vi "_ISV Calibration.vi"(6 "Progress Bar":refnum<vi>, 8 "Error In":errorcluster, 11 "ADC Channel Calibration In":string[][](table)) -> (0 "Error Out":errorcluster, 1 "aborted":bool, 2 "ADC Table":T1[](array[typedef]), 3 "ADC Channel Calibration Out":string[][](table))   [LabVIEW 2018]
uses:
  Type/_RT Configuration 2.ctl
  Type/_RT Command.ctl
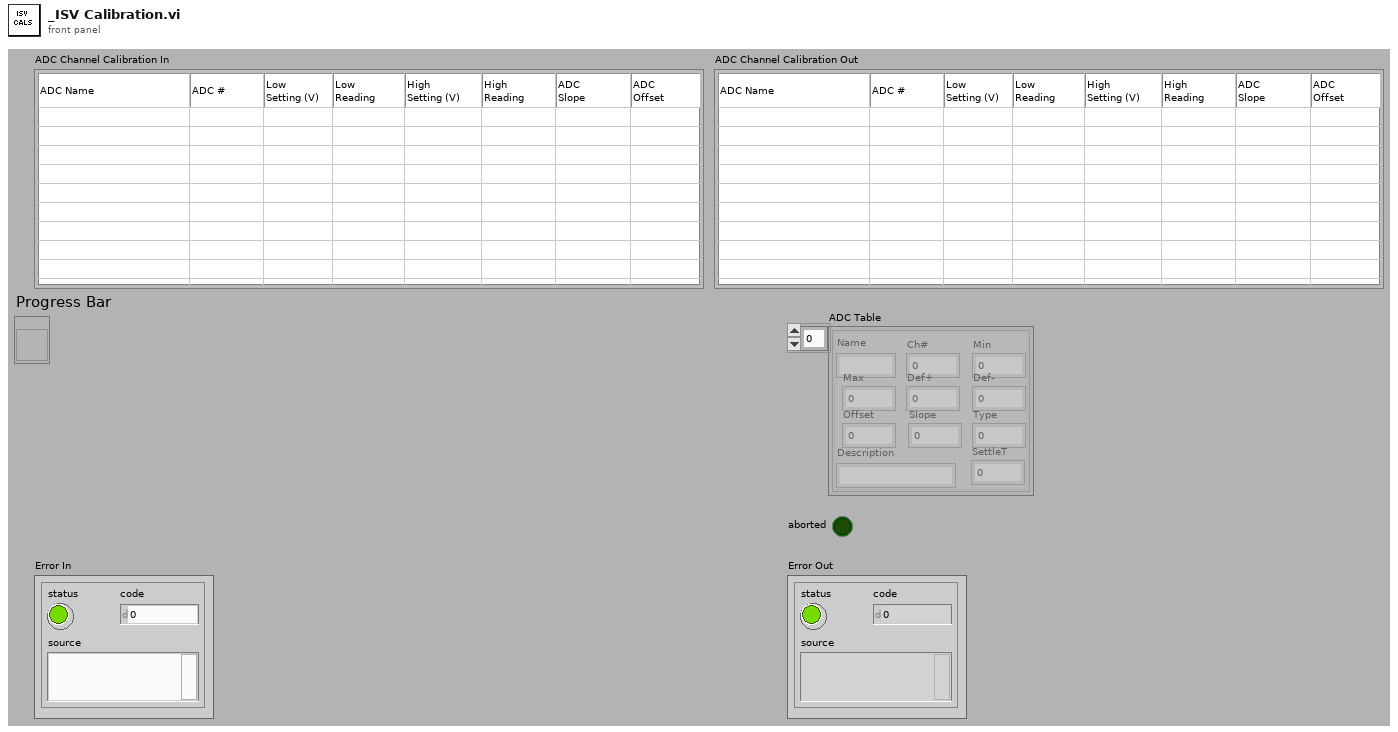
[diagram p1: front panel]
types:
  T1 = typedef "_RT Configuration 2.ctl" = cluster{"Name":string, "Ch#":u8, "Min":dbl, "Max":dbl, "Def+":dbl, "Def-":dbl, "Offset":dbl, "Slope":dbl, "Type":u8, "Description":string, "SettleT":dbl}
  T2 = typedef "_RT Command.ctl" = enum16{"xml Start Run", "xml Start Actual Run", "xml Stop Run", "xml Runtime Update", "xml Get Status", "xml Get Table", "xml Set Table", "xml Get Configuration", "xml System Status", "xml Set LC Input Logic", "xml Get Data", "xml Get Info", "Start", "StartActualRun", "Stop", "Runtime Update", "Get Data", "Get Info", "Get Status", "Get Param", "Get Config", "Get Table", "Read ADC", "Set Oscillator", "Update Config", "Update Table", "Set All Pol", "Set Pol and DC", "Set Max Mass", "Toggle RP", "Toggle EL", "Set PIC", "Initialize Turbo", "Send Turbo Comm", "Close Turbo", "P1", "P2", "P3", "Send Serial", "Set LC Out", "Get LC In", "Read VAC", "Test Table", "Toggle Power", "Get Startup", "Set Startup", "Get ADC Table", "Set ADC Table", "Get Brief Status", "Get Detail Status", "Auxiliary Update", "Set CC Logics", "Test Channel", "Set CC Input Logics", "Ignore Error", "invalid"}
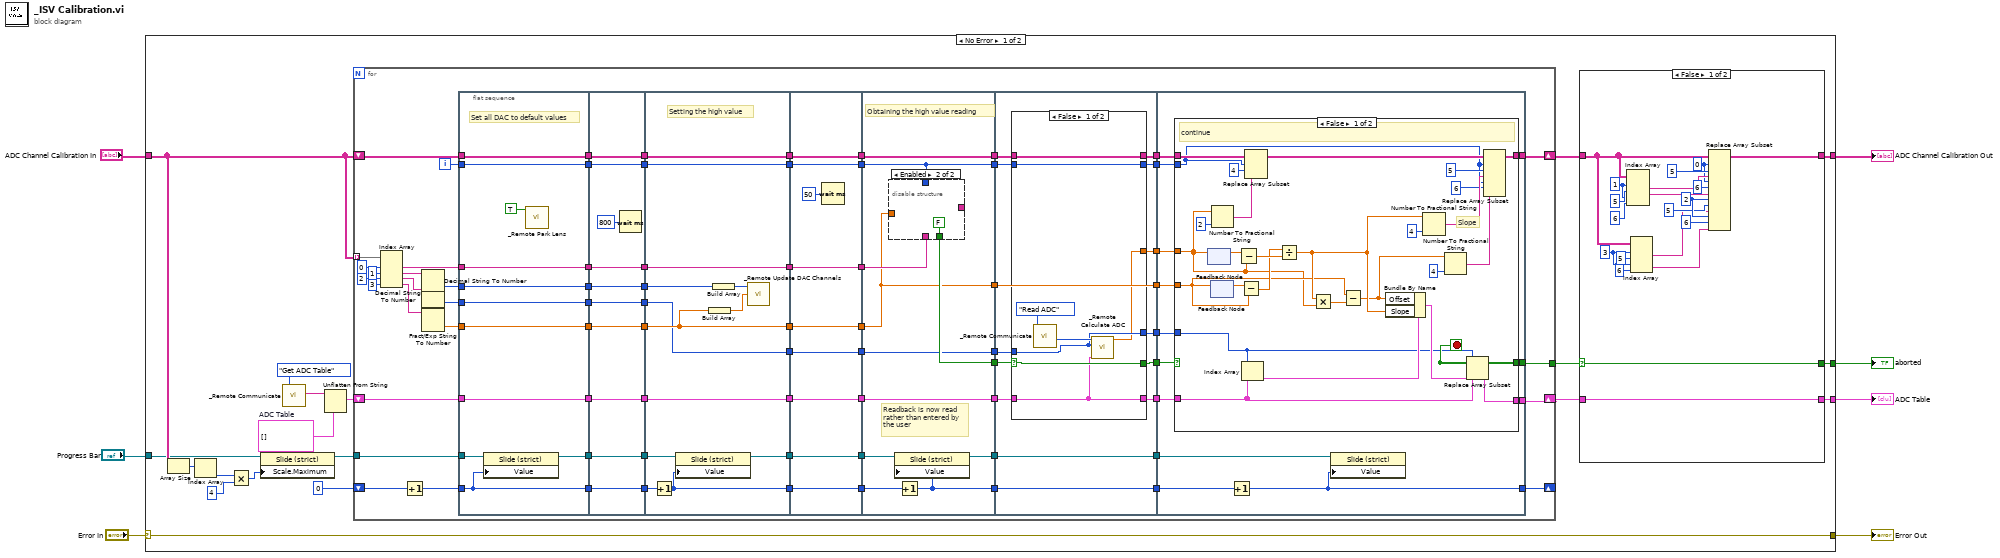
[diagram p0: block diagram]
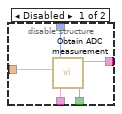
[diagram p2: hidden frame]
diagram:
  n1 = case shown="No Error" "Error In" {
    selector: "Error In" -> [w22 w253]
    tunnel: [w19 _] -> w7
    tunnel: [w21 w252] -> w6
    tunnel: "ADC Channel Calibration In" -> [w15 w252]
    tunnel: [w22 w253] -> w3
    tunnel: [w17 _] -> w2
    tunnel: "Progress Bar" -> [w13 _]
    frame No Error {
      w26 = T1[] []  # ADC Table
      n2 = Array Size(array=w15) -> (size(s)=w14:i32[])
      n3 = Index Array(array=w14) -> (element=w12:i32)  [unwired: 1 in]
      n4 = Multiply(x=w12, y=4) -> (x*y=w11:i32)
      n5 = property class="Slide (strict)"(reference=w13, "Scale.Maximum"=w11) -> (reference out=w9:refnum<vi>)  [unwired: 1 in, 1 out]
      n6 = call "_Remote Communicate.vi"("Command"=_RT_Command."Get ADC Table") -> ("Info"=w25:string)  [unwired: 5 in, 3 out]
      n7 = Unflatten From String(type=w26, binary string=w25) -> (value=w24:T1[])  [unwired: 1 in, 4 out]
      n8 = for {
        tunnel: w15 -> [w99] mode=indexing
        shift-right: [w96] -> w16
        shift-left: w15 -> [w97]
        tunnel: [w91] -> w20
        shift-right: [w93] -> w18
        shift-left: w24 -> [w92]
        tunnel: w9 -> [w42]
        shift-right: [w27] -> _
        shift-left: u8 0 ("Value") -> [w35]
        i -> [w98]
        stop <- w91 stop-if-true
        n9 = Index Array(array=w99, index #1=0 ("index"), index #2=1 ("index"), index #3=2 ("index"), index #4=3 ("index")) -> (element #1=w95:string, element #2=w94:string, element #3=w52:string, element #4=w53:string)
        n10 = Increment(x=w35) -> (x+1=w34:u8)
        n11 = Decimal String To Number(string=w94) -> (number=w60:i32)  [unwired: 3 out]
        n12 = Decimal String To Number(string=w52) -> (number=w46:i32)  [unwired: 3 out]
        n13 = Fract/Exp String To Number(string=w53) -> (number=w57:dbl)  [unwired: 4 out]
        n14 = flat-sequence {
          tunnel: [w109] -> w86
          tunnel: [w108] -> w84
          tunnel: [w110] -> w82
          tunnel: w97 -> [w110]
          tunnel: w95 -> [w108]
          tunnel: w98 -> [w109]
          tunnel: w92 -> [w107]
          tunnel: [w107] -> w80
          tunnel: [w105] -> w61
          tunnel: w60 -> [w105]
          tunnel: [w104] -> w58
          tunnel: w57 -> [w104]
          tunnel: [w103] -> w47
          tunnel: w46 -> [w103]
          tunnel: w42 -> [w102]
          tunnel: [w101] -> w40
          tunnel: w34 -> [w100]
          tunnel: [w100] -> w32
          tunnel: w86 -> [w120]
          tunnel: [w120] -> w85
          tunnel: w84 -> [w119]
          tunnel: [w119] -> w83
          tunnel: w82 -> [w118]
          tunnel: [w118] -> w81
          tunnel: w80 -> [w117]
          tunnel: [w117] -> w79
          tunnel: [w115] -> w62
          tunnel: w61 -> [w115]
          tunnel: [w114] -> w59
          tunnel: w58 -> [w114]
          tunnel: [w113] -> w48
          tunnel: w47 -> [w113]
          tunnel: [w112] -> w41
          tunnel: w40 -> [w112]
          tunnel: [w111] -> w33
          tunnel: w32 -> [w111]
          tunnel: [w132] -> w70
          tunnel: [w133] -> w68
          tunnel: [w131] -> w66
          tunnel: [w130] -> w64
          tunnel: w85 -> [w132]
          tunnel: w83 -> [w133]
          tunnel: w81 -> [w131]
          tunnel: w79 -> [w130]
          tunnel: w62 -> [w127]
          tunnel: w59 -> [w126]
          tunnel: [w126] -> w55
          tunnel: [w125] -> w49
          tunnel: w48 -> [w125]
          tunnel: w41 -> [w124]
          tunnel: [w123] -> w38
          tunnel: w33 -> [w122]
          tunnel: [w121] -> w30
          tunnel: w70 -> [w142]
          tunnel: [w142] -> w69
          tunnel: w68 -> [w141]
          tunnel: [w141] -> w67
          tunnel: w66 -> [w140]
          tunnel: [w140] -> w65
          tunnel: w64 -> [w139]
          tunnel: [w139] -> w63
          tunnel: [w137] -> w56
          tunnel: w55 -> [w137]
          tunnel: [w136] -> w50
          tunnel: w49 -> [w136]
          tunnel: [w135] -> w39
          tunnel: w38 -> [w135]
          tunnel: [w134] -> w31
          tunnel: w30 -> [w134]
          tunnel: w69 -> [w150]
          tunnel: w67 -> [w153]
          tunnel: w65 -> [w151]
          tunnel: [w151] -> w78
          tunnel: [w152] -> w76
          tunnel: [w150] -> w74
          tunnel: [w149] -> w72
          tunnel: w63 -> [w149]
          tunnel: w56 -> [w147]
          tunnel: [w148] -> w51
          tunnel: w50 -> [w148]
          tunnel: [w147] -> w43
          tunnel: w39 -> [w146]
          tunnel: [w145] -> w36
          tunnel: w31 -> [w144]
          tunnel: [w143] -> w28
          tunnel: w78 -> [w167]
          tunnel: [w173] -> w77
          tunnel: w76 -> [w171]
          tunnel: [w170] -> w75
          tunnel: w74 -> [w168]
          tunnel: [w169] -> w73
          tunnel: w72 -> [w172]
          tunnel: [w165] -> w71
          tunnel: [w166] -> w54
          tunnel: w51 -> [w164]
          tunnel: [w163] -> w45
          tunnel: [w162] -> w44
          tunnel: w43 -> [w162]
          tunnel: [w161] -> w37
          tunnel: w36 -> [w161]
          tunnel: [w160] -> w29
          tunnel: w28 -> [w160]
          tunnel: [w197] -> w96
          tunnel: w77 -> [w198]
          tunnel: w75 -> [w194]
          tunnel: w73 -> [w195]
          tunnel: w71 -> [w193]
          tunnel: [w192] -> w93
          tunnel: [w191] -> w91
          tunnel: w54 -> [w196]
          tunnel: w45 -> [w190]
          tunnel: w44 -> [w189]
          tunnel: w37 -> [w188]
          tunnel: w29 -> [w187]
          tunnel: [w186] -> w27
          frame #0 {
            # "Set all DAC to default values"
            n15 = property class="Slide (strict)"(reference=w102, "Value"=w100) -> (reference out=w101:refnum<vi>)  [unwired: 1 in, 1 out]
            n16 = call "_Remote Park Lens.vi"("All Ch (F)"=TRUE) -> ()  [unwired: 1 in, 6 out]
          }
          frame #1 {
            n17 = Wait (ms)(milliseconds to wait=u32 800) -> ()  [unwired: 1 out]
          }
          frame #2 {
            # "Setting the high value"
            n18 = Increment(x=w122) -> (x+1=w121:u8)
            n19 = property class="Slide (strict)"(reference=w124, "Value"=w121) -> (reference out=w123:refnum<vi>)  [unwired: 1 in, 1 out]
            n20 = Build Array(w126) -> (w128:dbl[])
            n21 = Build Array(w127) -> (w129:i32[])
            n22 = call "_Remote Update DAC Channels.vi"("UserValue"=w128, "Ch#"=w129) -> ()  [unwired: 1 in, 2 out]
          }
          frame #3 {
            n23 = Wait (ms)(milliseconds to wait=u32 50) -> ()  [unwired: 1 out]
          }
          frame #4 {
            # "Readback is now read\nrather than entered by\nthe user"
            # "Obtaining the high value reading"
            n24 = disable-structure shown="Enabled" {
              disable-tunnel: w153 -> [w158 _]
              disable-tunnel: [w157 _] -> _
              disable-tunnel: [w156 FALSE ("Aborted")] -> w152
              disable-tunnel: w150 -> [w155 _]
              disable-tunnel: w147 -> [w154 _]
              frame Disabled {
                n25 = call "Obtain ADC measurement.vi"("index"=w155, "Expected Reading"=w154, "DAC Channel Name"=w158) -> ("Aborted"=w156:bool, "Reading"=w157:string)  [unwired: 3 in]
              }
              frame Enabled {
              }
            }
            n26 = Increment(x=w144) -> (x+1=w143:u8)
            n27 = property class="Slide (strict)"(reference=w146, "Value"=w143) -> (reference out=w145:refnum<vi>)  [unwired: 1 in, 1 out]
          }
          frame #5 {
            n28 = case shown="False" w171 {
              selector: w171 -> [w179 _]
              tunnel: [w174 _] -> w173
              tunnel: w172 -> [w176 w183]
              tunnel: [w179 _] -> w170
              tunnel: [w178 w184] -> w169
              tunnel: w168 -> [w178 w184]
              tunnel: w167 -> [w177 w185]
              tunnel: [w177 w185] -> w166
              tunnel: [w176 w183] -> w165
              tunnel: w164 -> [w175 w182]
              tunnel: [w175 w182] -> w163
              frame False {
                n29 = call "_Remote Communicate.vi"("Command"=_RT_Command."Read ADC") -> ("Data Array"=w181:i32[])  [unwired: 5 in, 3 out]
                n30 = call "_Remote Calculate ADC.vi"("ADC Table"=w176, "ADC Channel (64)"=w175, "ADC Values"=w181) -> ("Raw Reading"=w174:dbl)  [unwired: 1 in, 3 out]
              }
              frame True {
              }
            }
          }
          frame #6 {
            n31 = case shown="False" w194 {
              selector: w194 -> [_ w226]
              tunnel: w198 -> [w199 _]
              tunnel: [w222 w228] -> w197
              tunnel: w196 -> [w217 w228]
              tunnel: w195 -> [w202 _]
              tunnel: w193 -> [w219 w227]
              tunnel: [w218 w227] -> w192
              tunnel: [_ w226] -> w191
              tunnel: w190 -> [w214 _]
              tunnel: w189 -> [w200 _]
              frame False {
                # "Slope"
                # "continue"
                n32 = feedback-in #1(w199) -> ()
                n33 = feedback #1() -> (w212:dbl)  [unwired: 1 in]
                n34 = feedback #2() -> (w211:dbl)  [unwired: 1 in]
                n35 = feedback-in #2(w200) -> ()
                n36 = Number To Fractional String(number=w199, precision (6)=i16 2) -> (F-format string=w213:string)  [unwired: 2 in]
                n37 = Subtract(x=w212, y=w199) -> (x-y=w210:dbl)
                n38 = Subtract(x=w211, y=w200) -> (x-y=w209:dbl)
                n39 = Index Array(array=w219, index=w214) -> (element=w216:T1)
                n40 = Replace Array Subset(array=w217, new element=w213, index (row)=w202, index (col)=4 ("disabled index (col)")) -> (w220:string[][])
                n41 = Divide(x=w209, y=w210) -> (x/y=w208:dbl)
                n42 = Multiply(x=w208, y=w199) -> (x*y=w207:dbl)
                n43 = Subtract(x=w200, y=w207) -> (x-y=w204:dbl)
                n44 = Bundle By Name(cluster=w216, "Offset"=w204, "Slope"=w208) -> (w215:T1)
                n45 = Number To Fractional String(number=w208, precision (6)=i16 4) -> (F-format string=w223:string)  [unwired: 2 out]
                n46 = Number To Fractional String(number=w204, precision (6)=i16 4) -> (F-format string=w203:string)  [unwired: 2 out]
                n47 = Replace Array Subset(array=w219, new element=w215, index=w214) -> (w218:T1[])
                n48 = Replace Array Subset(array=w220, new element #1=w223, index (row) #1=w202, index (col) #1=5 ("disabled index (col)"), new element #2=w203, index (row) #2=w202, index (col) #2=6 ("index (row)")) -> (w222:string[][])
              }
              frame True {
                # "Previous Step Aborted"
              }
            }
            n49 = Increment(x=w187) -> (x+1=w186:u8)
            n50 = property class="Slide (strict)"(reference=w188, "Value"=w186) -> ()  [unwired: 1 in, 2 out]
          }
        }
      }
      n51 = case shown="False" w20 {
        selector: w20 -> [w248 w250]
        tunnel: [w244 w251] -> w21
        tunnel: w16 -> [w237 w251]
        tunnel: [w248 w250] -> w19
        tunnel: w18 -> [w247 w249]
        tunnel: [w247 w249] -> w17
        frame False {
          w233 = 2 ("index (row)")
          w235 = 3 ("index (row)")
          w239 = 0 ("index (row)")
          w238 = 1 ("index (row)")
          n52 = Index Array(array=w237, index (row) #1=w238, index (col) #1=5 ("disabled index (col)"), index (row) #2=w238, index (col) #2=6 ("disabled index (col)")) -> (element #1=w242:string, element #2=w240:string)
          n53 = Index Array(array=w237, index (row) #1=w235, index (col) #1=5 ("disabled index (col)"), index (row) #2=w235, index (col) #2=6 ("disabled index (col)")) -> (element #1=w229:string, element #2=w230:string)
          n54 = Replace Array Subset(array=w237, new element #1=w242, index (row) #1=w239, index (col) #1=5 ("disabled index (col)"), new element #2=w240, index (row) #2=w239, index (col) #2=6 ("disabled index (col)"), new element #3=w229, index (row) #3=w233, index (col) #3=5 ("disabled index (col)"), new element #4=w230, index (row) #4=w233, index (col) #4=6 ("disabled index (col)")) -> (w244:string[][])
        }
        frame True {
        }
      }
    }
    frame Error {
    }
  }
  "aborted" <- w7
  "ADC Channel Calibration Out" <- w6
  "Error Out" <- w3
  "ADC Table" <- w2
